vi "Read Enum Reference.vi"(8 "error in (no error)":errorcluster, 11 "List Box Enum Column in":refnum<class "List Box Enum Column.lvclass">) -> (0 "error out":errorcluster, 2 "Enum Reference":refnum<vi>, 3 "List Box Enum Column out":refnum<class "List Box Enum Column.lvclass">)   [LabVIEW 2013, in "Table Manager.lvlib" / "List Box Enum Column.lvclass"]
uses:
  List Box Enum Column.lvclass
  <vilib>/NI/Tag Bus/tag/Data Type.ctl
  List Box Enum Column.lvclass/List Box Enum Column.ctl
  <vilib>/NI/Tag Bus/tag/tag descriptor.lvclass
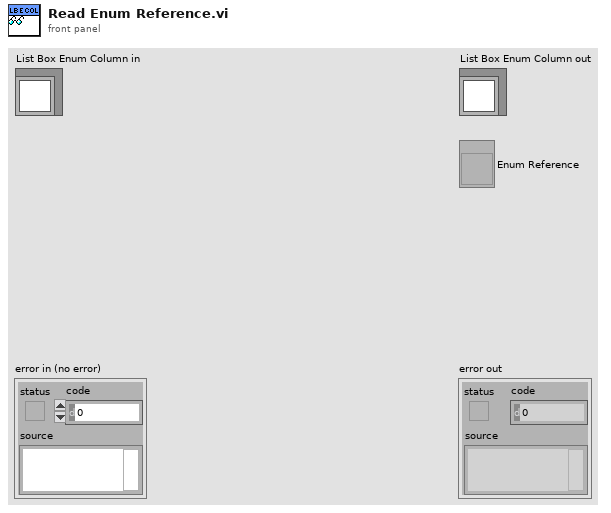
[diagram p1: front panel]
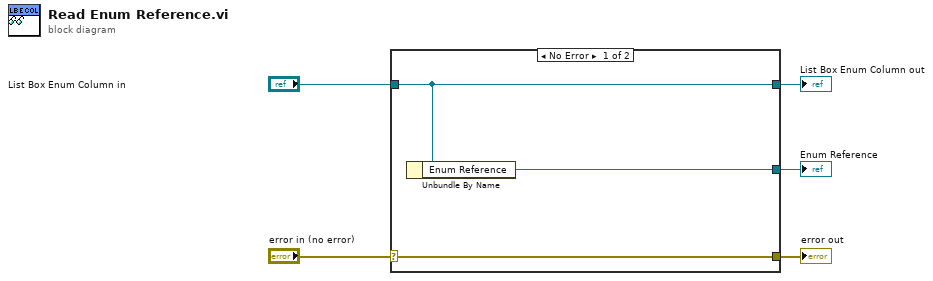
[diagram p0: block diagram]
diagram:
  n1 = case shown="No Error" "error in (no error)" {
    selector: "error in (no error)" -> [w8 w9]
    tunnel: [w8 w9] -> w4
    tunnel: [w7 w10] -> w2
    tunnel: "List Box Enum Column in" -> [w7 w10]
    tunnel: [w6 _] -> w1
    frame No Error {
      n2 = Unbundle By Name(w7) -> ("Enum Reference"=w6:refnum<vi>)
    }
    frame Error {
    }
  }
  "error out" <- w4
  "List Box Enum Column out" <- w2
  "Enum Reference" <- w1
